vi "textToSpeech.vi"() -> ()   [LabVIEW 2021]
uses:
  System.Speech
panel:
  in  "String":string
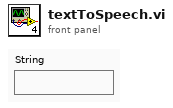
[diagram p1: front panel]
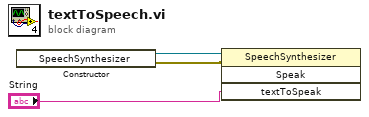
[diagram p0: block diagram]
diagram:
  n1 = constructor class="SpeechSynthesizer"() -> (reference out=w3:refnum<k24>, error out=w2:errorcluster)  [unwired: 3 in, 1 out]
  n2 = invoke class="SpeechSynthesizer" method="Speak"(reference=w3, error in=w2, "textToSpeak"="String") -> ()  [unwired: 1 in, 4 out]
